vi "Lift Controller.vi"(8 "error in":errorcluster) -> ()   [LabVIEW 2019]
doc: "This VI executes continuously carrying out the current operation and responding to updates or new operations. It will often contain the timing or control code that is difficult to place directly in TeleOp. This VI generally opens all sensors and motors and isolates the rest of the robot code from knowing how the operations are carried out."
uses:
  <vilib>/Rock Robotics/WPI/Framework/Completion Status.ctl
  Lift Setpoints.ctl
  Lift Operations.ctl
  <vilib>/Rock Robotics/WPI/SafetyOutput/WPI_SafetyOutputConfigMenu.ctl
  <vilib>/Rock Robotics/WPI/ThirdParty/REV Robotics/SPARK MAX/Typedef/Spark MAX Control Type.ctl
  <vilib>/Rock Robotics/Network Tables/NT Write Boolean.vi
panel:
  out "Setpoints":T1(graph)
  in  "Interactive Values":T2
  out "Current\nCmd":string
  in  "Buttons":cluster{"Execute Cmd":bool, "Abort Cmd":bool}
  out "Command Timing":cluster{"Start Time (ms)":u32, "Iterations":i32}
  out "Status":T4
  # "Tip: It may be helpful to observe inputs and sensor values.\nYou may also want to display tuning or debugging controls."
  # "Interactive Command: You may fill in the settings for a command\nand schedule it with the Execute button. You can observe and abort\nany command while fine tuning the code for the controller."
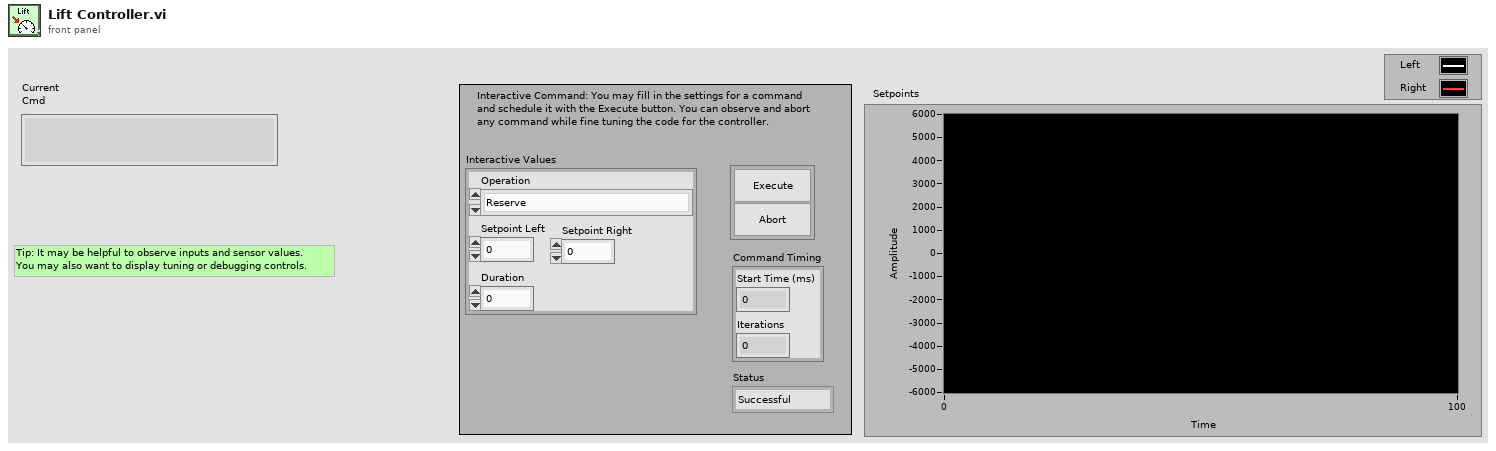
[diagram p1: front panel]
types:
  T1 = cluster{"Left Setpoint":dbl, "Right Setpoint":dbl}
  T2 = typedef "Lift Setpoints.ctl" = cluster{"Operation":T3, "Setpoint Left":dbl, "Duration":dbl, "Setpoint Right":dbl}
  T3 = typedef "Lift Operations.ctl" = enum16{"Reserve", "Read Current", "Immediate"}
  T4 = typedef "Completion Status.ctl" = enum16{"Successful", "Aborted", "Incomplete"}
  T5 = typedef "WPI_SafetyOutputConfigMenu.ctl" = enum16{"Enable", "Disable"}
  T6 = typedef "WPI_MotorControlDeviceRef.ctl" = cluster{"DeviceStatus":errorcluster, "Type":T7, "PWM":cluster{"PWM Channel":T8, "DeadBand":T9}, "CAN":cluster{"Device Number":u8, "SetOutput VI Ref":variant, "GetOutput VI Ref":variant, "Enable VI Ref":variant, "Disable VI Ref":variant, "Data":variant}, "Invert":bool, "DIO PWM":cluster{"PWM \"Enable\" Channel":T8, "DIOChannel":T10, "PWM Rate":dbl}}
  T7 = typedef "WPI_MotorControlType.ctl" = enum16{"PWM", "CAN", "DIO PWM"}
  T8 = typedef "FPGA_DIOPWMChannel.ctl" = enum8{"PWM 0", "PWM 1", "PWM 2", "PWM 3", "PWM 4", "PWM 5", "PWM 6", "PWM 7", "PWM 8", "PWM 9", "PWM MXP 0", "PWM MXP 1", "PWM MXP 2", "PWM MXP 3", "PWM MXP 4", "PWM MXP 5", "PWM MXP 6", "PWM MXP 7", "PWM MXP 8", "PWM MXP 9", "Invalid"}
  T9 = typedef "WPI_PWMDeadband.ctl" = cluster{"Name":string, "maxPositivePwm":i32, "minPositivePwm":i32, "centerPwm":i32, "maxNegativePwm":i32, "minNegativePwm":i32, "angularRange":u16}
  T10 = typedef "FPGA_DIOChannel.ctl" = enum8{"DIO 0", "DIO 1", "DIO 2", "DIO 3", "DIO 4", "DIO 5", "DIO 6", "DIO 7", "DIO 8", "DIO 9", "DIO MXP 0", "DIO MXP 1", "DIO MXP 2", "DIO MXP 3", "DIO MXP 4", "DIO MXP 5", "DIO MXP 6", "DIO MXP 7", "DIO MXP 8", "DIO MXP 9", "DIO MXP 10", "DIO MXP 11", "DIO MXP 12", "DIO MXP 13", "DIO MXP 14", "DIO MXP 15", "SPI Port CS1", "SPI Port CS2", "SPI Port CS3", "SPI Port MISO", "SPI Port MOSI", "Invalid"}
  T11 = typedef "Command Status Info.ctl" = cluster{"Name":string, "Status":T4, "notifier out":T12}
  T12 = typedef "Completion Notifier.ctl" = refnum<notifier>
  T13 = cluster{"Current Command":T2, "Command Timing":cluster{"Start Time (ms)":u32, "Iterations":i32}, "Command Arguments":cluster{"Command Info":T11, "Description":string, "Default Command":T2, "queue out":refnum<queue>, "Subsystem Name":string}}
  T14 = typedef "Spark MAX Control Type.ctl" = enum16{"Percent VBus", "Voltage", "Velocity", "Position", "Smart Motion", "Current", "Smart Velocity"}
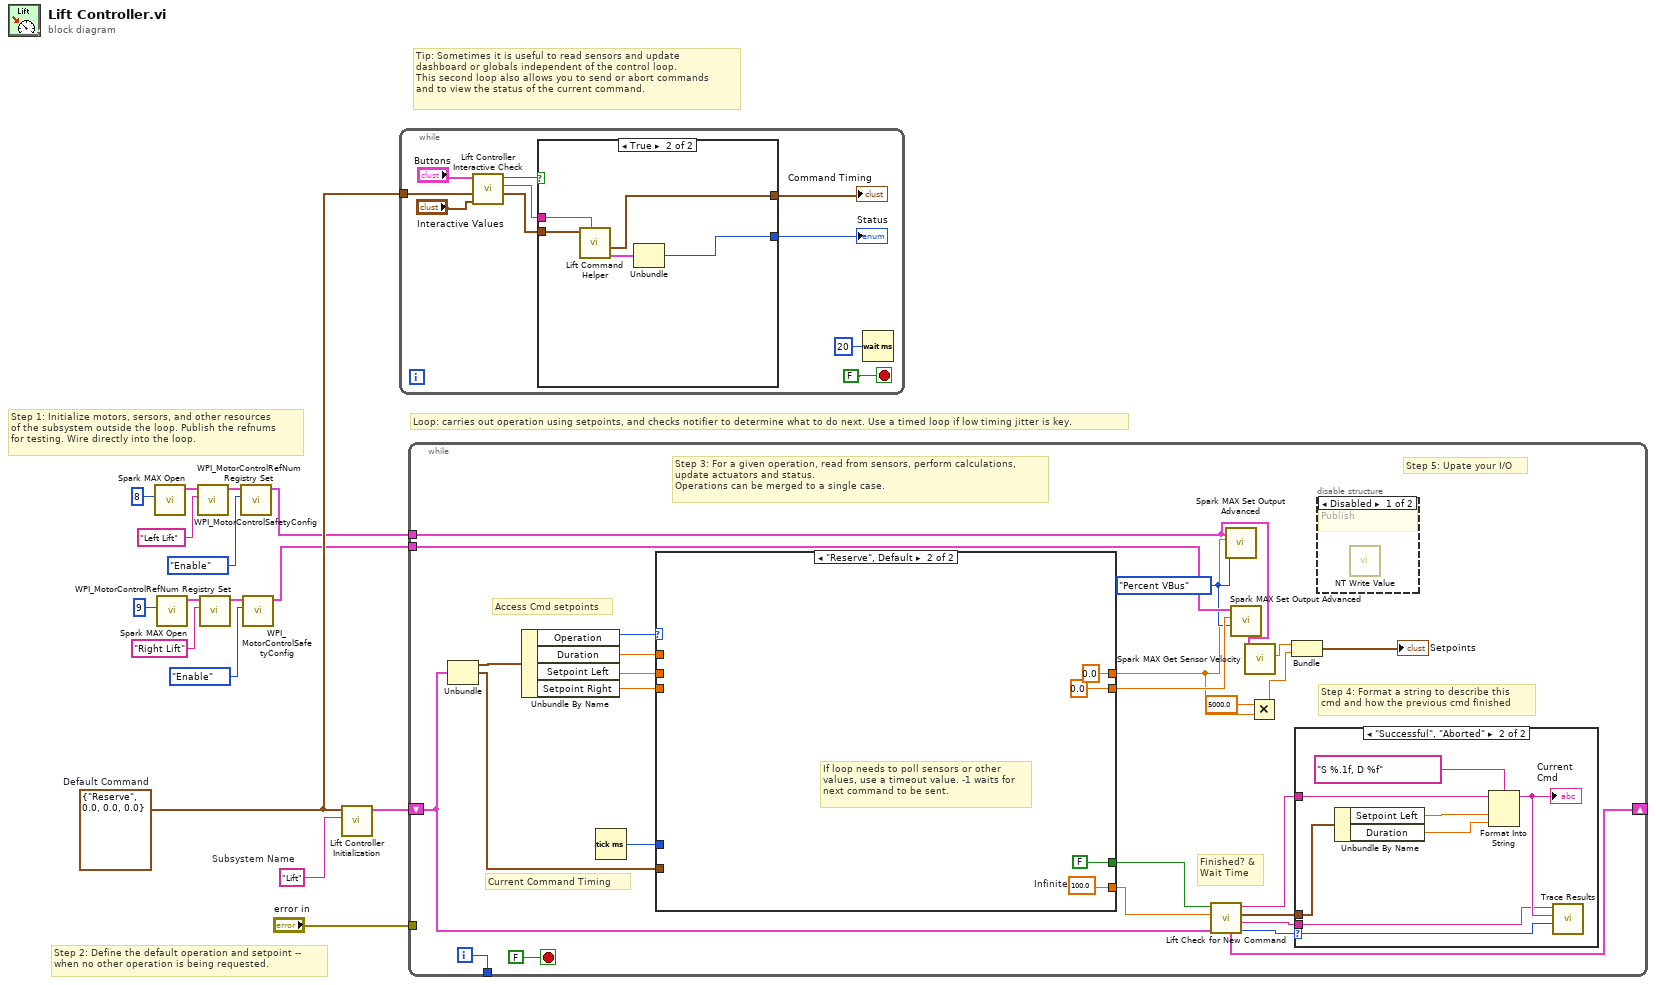
[diagram p0: block diagram]
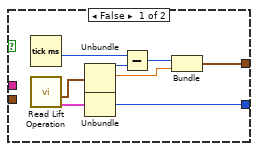
[diagram p2: hidden frame]
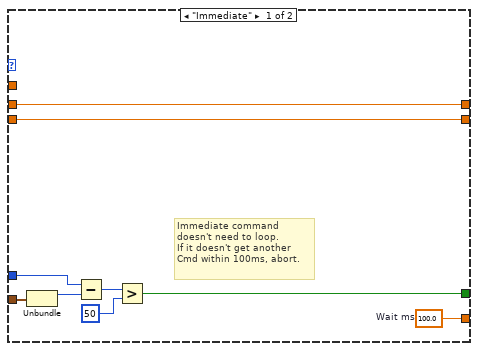
[diagram p5: hidden frame]
diagram:
  w13 = T2 {"Operation"=enum."Reserve", "Setpoint Left"=0.0, "Duration"=0.0, "Setpoint Right"=0.0}  # Default Command
  w14 = "Lift"  # Subsystem Name
  # "Tip: Sometimes it is useful to read sensors and update\ndashboard or globals independent of the control loop.\nThis second loop also allows you to send or abort commands\nand to view the status of the current command."
  # "Step 2: Define the default operation and setpoint --\nwhen no other operation is being requested."
  # "Step 1: Initialize motors, sersors, and other resources\nof the subsystem outside the loop. Publish the refnums\nfor testing. Wire directly into the loop."
  # "Loop: carries out operation using setpoints, and checks notifier to determine what to do next. Use a timed loop if low timing jitter is key."
  n1 = call <vilib>:"Spark MAX Open.vi"("Device Number"=u8 8) -> ("MotorControlDeviceRef"=w4:T6)  [unwired: 9 in, 1 out]
  n2 = call <vilib>:"Spark MAX Open.vi"("Device Number"=u8 9) -> ("MotorControlDeviceRef"=w6:T6)  [unwired: 9 in, 1 out]
  n3 = call <vilib>:"WPI_MotorControlRefNum Registry Set.vi"("refnum name"="Left Lift", "MotorControlDevRef"=w4) -> ("MotorControlDevRef"=w3:T6)  [unwired: 8 in, 1 out]
  n4 = call <vilib>:"WPI_MotorControlRefNum Registry Set.vi"("refnum name"="Right Lift", "MotorControlDevRef"=w6) -> ("MotorControlDevRef"=w5:T6)  [unwired: 8 in, 1 out]
  n5 = call <vilib>:"WPI_MotorControlSafetyConfig.vi"("mode"=WPI_SafetyOutputConfigMenu."Enable", "MotorControlDevRef"=w3) -> ("MotorControlDevRef"=w12:T6)  [unwired: 8 in, 1 out]
  n6 = call <vilib>:"WPI_MotorControlSafetyConfig.vi"("mode"=WPI_SafetyOutputConfigMenu."Enable", "MotorControlDevRef"=w5) -> ("MotorControlDevRef"=w11:T6)  [unwired: 8 in, 1 out]
  n7 = call "Lift Controller Initialization.vi"("Subsystem Name"=w14, "Default Command"=w13) -> ("Current Command"=w15:T13)  [unwired: 9 in]
  n8 = while {
    tunnel: w13 -> [w23]
    stop <- FALSE stop-if-true
    n9 = call "Lift Controller Interactive Check.vi"("Interactive Command in"="Interactive Values", "Default Command"=w23, "Buttons"="Buttons") -> ("Interactive Command out"=w20:T2, "Trace String"=w21:string, "Schedule"=w22:bool)  [unwired: 6 in]
    n10 = case shown="True" w22 {
      tunnel: [w34 w39] -> w19
      tunnel: w20 -> [_ w37]
      tunnel: [w30 w35] -> w18
      tunnel: w21 -> [_ w38]
      frame False {
        n11 = Tick Count (ms)() -> (millisecond timer value=w29:u32)
        n12 = call "Read Lift Operation.vi"() -> ("Command Info"=w27:T11, "SubSystem Data"=w28:T2)  [unwired: 9 in, 1 out]
        n13 = Unbundle(w28) -> ("Operation"=w33:T3, "Setpoint Left"=w31:dbl)  [unwired: 2 out]
        n14 = Unbundle(w27) -> ("Status"=w34:T4)  [unwired: 2 out]
        n15 = Subtract(x=w29, y=w33) -> (x-y=w32:u32)
        n16 = Bundle(w32, "Setpoint Left"=w31) -> (w30:cluster{u32, "Setpoint Left":dbl})  [unwired: 1 in]
      }
      frame True {
        n17 = call "Lift Command Helper.vi"("Description"=w38, "SubSystem Data"=w37) -> ("Command Info Out"=w36:T11, "Command Timing"=w35:cluster{"Start Time (ms)":u32, "Iterations":i32})  [unwired: 7 in, 1 out]
        n18 = Unbundle(w36) -> ("Status"=w39:T4)  [unwired: 2 out]
      }
    }
    "Status" <- w19
    "Command Timing" <- w18
    n19 = Wait (ms)(milliseconds to wait=u32 20) -> ()  [unwired: 1 out]
  }
  n20 = while {
    shift-right: [w57] -> _
    shift-left: w15 -> [w50]
    tunnel: [w64] -> _
    tunnel: "error in" -> [_]
    tunnel: w12 -> [w43]
    tunnel: w11 -> [w48]
    i -> [w64]
    stop <- FALSE stop-if-true
    w46 = Spark_MAX_Control_Type."Percent VBus" ("Control Mode")
    # "Step 5: Upate your I/O"
    # "Step 4: Format a string to describe this\ncmd and how the previous cmd finished"
    # "Current Command Timing"
    # "Access Cmd setpoints"
    # "Finished? &\nWait Time"
    # "Step 3: For a given operation, read from sensors, perform calculations,\nupdate actuators and status.\nOperations can be merged to a single case."
    n21 = Unbundle(w50) -> ("Current Command"=w63:T2, "Command Timing"=w59:cluster{"Start Time (ms)":u32, "Iterations":i32})  [unwired: 1 out]
    n22 = Unbundle By Name(w63) -> ("Operation"=w62:T3, "Duration"=w61:dbl, "Setpoint Left"=w58:dbl, "Setpoint Right"=w49:dbl)
    n23 = Tick Count (ms)() -> (millisecond timer value=w60:u32)
    n24 = case shown="\"Reserve\", Default" w62 {
      tunnel: [w82 w86] -> w55
      tunnel: [w76 FALSE ("ignore previous (F)")] -> w56
      tunnel: w59 -> [w78 _]
      tunnel: w61 -> [_ _]
      tunnel: w60 -> [w77 _]
      tunnel: w58 -> [w75 _]
      tunnel: w49 -> [w74 _]
      tunnel: [w75 0.0 ("Setpoint Left")] -> w42
      tunnel: [w74 0.0 ("Setpoint Right")] -> w47
      frame "Immediate" {
        w82 = 100.0  # Wait ms
        # "Immediate command\ndoesn't need to loop.\nIf it doesn't get another\nCmd within 100ms, abort."
        n25 = Unbundle(w78) -> ("Start Time (ms)"=w81:u32)  [unwired: 1 out]
        n26 = Subtract(x=w77, y=w81) -> (x-y=w80:u32)
        n27 = Greater?(x=w80, y=u8 50 ("Left Motor")) -> (0:w76:bool)
      }
      frame "Reserve", Default {
        w86 = 100.0  # Infinite
        # "If loop needs to poll sensors or other\nvalues, use a timeout value. -1 waits for\nnext command to be sent."
      }
    }
    n28 = call "Lift Check for New Command.vi"("Current Command"=w50, "Wait time (ms)"=w55, "Finished?"=w56) -> ("Completion"=w51:T4, "Subsystem Name"=w52:string, "Current Command"=w53:T2, "Initial Trace String"=w54:string, "NextCommand"=w57:T13)  [unwired: 4 in]
    n29 = call <vilib>:"Spark MAX Set Output Advanced.vi"("Control Mode"=w46, "Setpoint"=w42, "MotorControlDevRef"=w43) -> ()  [unwired: 7 in, 2 out]
    n30 = call <vilib>:"Spark MAX Set Output Advanced.vi"("Control Mode"=w46, "Setpoint"=w47, "MotorControlDevRef"=w48) -> ()  [unwired: 7 in, 2 out]
    n31 = call <vilib>:"Spark MAX Get Sensor Velocity.vi"("MotorControlDevRef in"=w43) -> ("Sensor Velocity"=w44:dbl)  [unwired: 7 in, 3 out]
    n32 = Multiply(x=5000.0, y=w42) -> (x*y=w41:dbl)
    n33 = Bundle("Sensor Velocity"=w44, w41) -> (→"Setpoints":cluster{"Sensor Velocity":dbl, dbl})  [unwired: 1 in]
    n34 = case shown="\"Successful\", \"Aborted\"" w51 {
      selector: w51 -> [_ w73]
      tunnel: w54 -> [_ w69]
      tunnel: w53 -> [_ w70]
      tunnel: w52 -> [_ w66]
      frame "Incomplete", Default {
        # "Continuing current command"
      }
      frame "Successful", "Aborted" {
        # "Report and setup for next command"
        n35 = Unbundle By Name(w70) -> ("Setpoint Left"=w72:dbl, "Duration"=w67:dbl)
        n36 = Format Into String(format string="S %.1f, D %f", initial string=w69, w72, w67) -> (resulting string=w68:string)  [unwired: 1 in, 1 out]
        "Current\nCmd" <- w68
        n37 = call <vilib>:"Trace Results.vi"("Status of previous command"=w73, "Description"=w68, "Subsystem"=w66) -> ()  [unwired: 9 in]
      }
    }
    n38 = disable-structure shown="Disabled" {
      frame Disabled {
        # "Publish"
        n39 = call-poly <vilib>:"NT Write Value.vi"() -> ()  [unwired: 11 in, 1 out]
      }
      frame Enabled {
      }
    }
  }
